vi "Deinitialize.vi"(9 "VISA resource name":refnum<visa-resource-name>) -> (0 "error out":errorcluster)   [LabVIEW 2023, in "Aim TTi 1908P DMM.lvlib"]
uses:
  Aim TTi 1908P DMM.lvlib
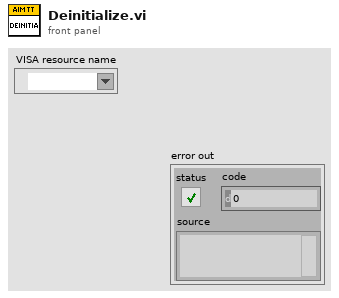
[diagram p1: front panel]
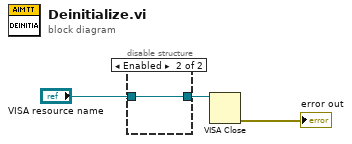
[diagram p0: block diagram]
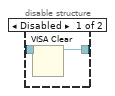
[diagram p2: hidden frame]
diagram:
  n1 = disable-structure shown="Enabled" {
    disable-tunnel: [w5 w6] -> w3
    disable-tunnel: "VISA resource name" -> [w4 w6]
    frame Disabled {
      n2 = VISA Clear(VISA resource name=w4) -> (VISA resource name out=w5:refnum<visa-resource-name>)  [unwired: 1 in, 1 out]
    }
    frame Enabled {
    }
  }
  n3 = VISA Close(VISA resource name=w3) -> (error out=→"error out":errorcluster)  [unwired: 1 in]
